vi "tm_getrecorderstatus.vi"(8 "error in (no error)":errorcluster, 11 "Handle":u32) -> (0 "error out":errorcluster, 1 "Count":i32, 2 "Index":i32, 3 "Handle":u32)   [LabVIEW 2015]
uses:
  tmcamcon.dll
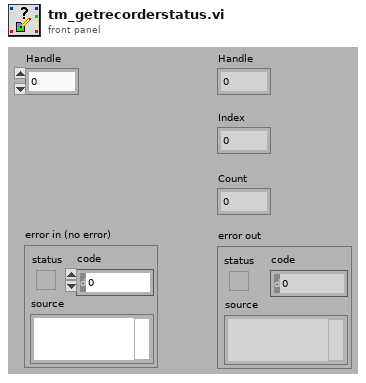
[diagram p1: front panel]
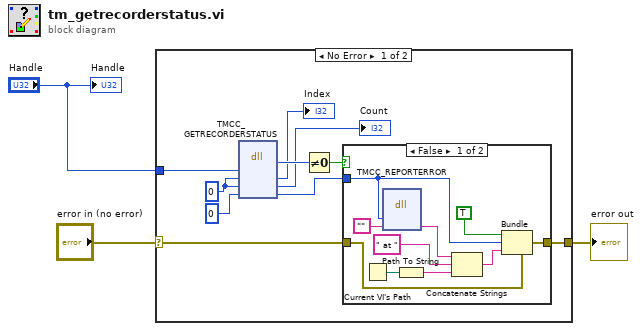
[diagram p0: block diagram]
diagram:
  n1 = case shown="No Error" "error in (no error)" {
    selector: "error in (no error)" -> [w9 w25]
    tunnel: [w8 w25] -> w2
    tunnel: "Handle" -> [w7 _]
    frame No Error {
      w6 = 0 ("totalframes")
      n2 = dll-call lib="tmcamcon.dll" fn="TMCC_GETRECORDERSTATUS"("handle"=w7, "index"=w6, "count"=w6, "Erval"=0) -> ("return type"=w13:u32, "index"=→"Index":i32, "count"=→"Count":i32, "Erval"=w11:i32)  [unwired: 4 in, 2 out]
      n3 = Not Equal To 0?(x=w13) -> (x != 0?=w10:bool)
      n4 = case shown="False" w10 {
        tunnel: w9 -> [w23 w24]
        tunnel: [w22 w24] -> w8
        tunnel: w11 -> [w16 _]
        frame False {
          n5 = Current VI's Path() -> (path=w21:path)
          n6 = dll-call lib="tmcamcon.dll" fn="TMCC_REPORTERROR"("error"=w16, "buf"="") -> ("buf"=w15:string)  [unwired: 5 in, 2 out]
          n7 = Path To String(path=w21) -> (string=w17:string)
          n8 = Concatenate Strings(w15, " at ", w17) -> (w20:string)
          n9 = Bundle(cluster=w23, "status"=TRUE, "code"=w16, "source"=w20) -> (w22:errorcluster)
        }
        frame True {
        }
      }
    }
    frame Error {
    }
  }
  "error out" <- w2
  "Handle" <- "Handle"
